vi "dfd_Normalization 2D.vi"(10 "scale type":T1, 11 "2D Array (col-major)":dbl[][](array[numeric])) -> (3 "max norm":dbl)   [LabVIEW 2017, in "NI_DigFilterLicensed.lvlib"]
uses:
  <vilib>/addons/Digital Filter Design/NI_DigFilterLicensed.lvlib
  <vilib>/addons/Digital Filter Design/_Objects.llb/DFD Coef Norm Type.ctl
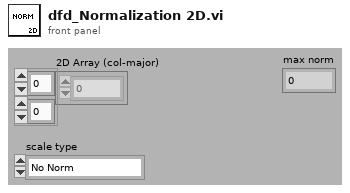
[diagram p1: front panel]
types:
  T1 = typedef "NI_DigFilterLicensed.lvlib/DFD Coef Norm Type.ctl" = enum16{"No Norm", "Time Domain 1-Norm", "Time Domain 2-Norm", "Time Domain Inf-Norm"}
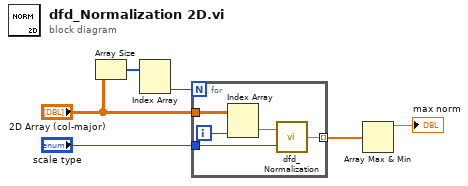
[diagram p0: block diagram]
diagram:
  n1 = Array Size(array="2D Array (col-major)") -> (size(s)=w3:i32[])
  n2 = Index Array(array=w3) -> (element #2=w2:i32)  [unwired: 2 in, 1 out]
  n3 = for {
    N: w2 -> [_]
    tunnel: "scale type" -> [w11]
    tunnel: [w10] -> w6 mode=indexing
    tunnel: "2D Array (col-major)" -> [w9]
    i -> [w8]
    n4 = Index Array(array=w9, index (col)=w8) -> (element=w7:dbl[])  [unwired: 1 in]
    n5 = call <vilib>:"dfd_Normalization.vi"("scale type"=w11, "h(n)"=w7) -> ("norm"=w10:dbl)
  }
  n6 = Array Max & Min(array=w6) -> (max value=→"max norm":dbl)  [unwired: 3 out]
